vi "Backward Bracket Search.VI"(0 "string input with brackets":string) -> (1 "string start":string, 2 "string rest":string)   [LabVIEW 2010, in "NI_Gmath.lvlib"]
uses:
  NI_Gmath.lvlib
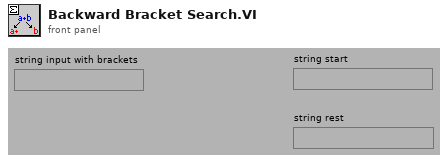
[diagram p1: front panel]
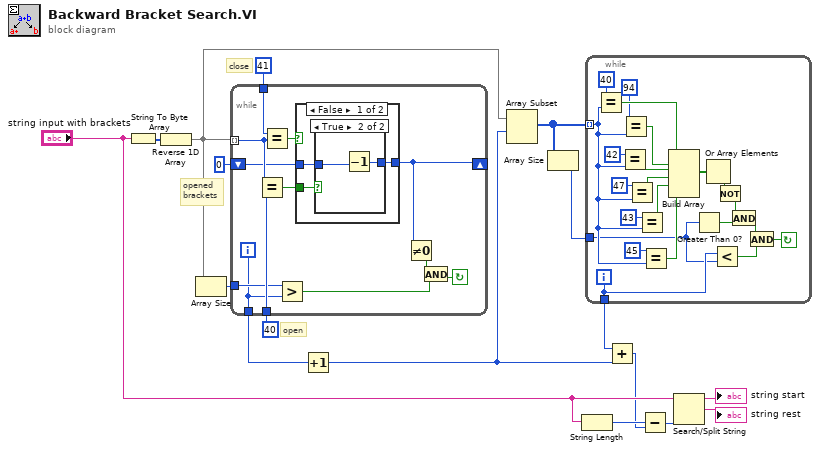
[diagram p0: block diagram]
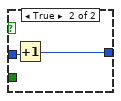
[diagram p3: hidden frame]
diagram:
  # "open"
  # "close"
  # "opened\nbrackets"
  n1 = String To Byte Array(string="string input with brackets") -> (unsigned byte array=w14:u8[])
  n2 = Reverse 1D Array(array=w14) -> (reversed array=w4:u8[])
  n3 = Array Size(array=w4) -> (size(s)=w13:i32)
  n4 = while {
    tunnel: [w18] -> w12
    tunnel: w13 -> [w23]
    tunnel: 40 -> [w27]
    tunnel: 41 -> [w29]
    tunnel: w4 -> [w26] mode=indexing
    shift-left: 0 -> [w20]
    shift-right: [w24] -> _
    i -> [w18]
    stop <- w21 continue-if-true
    n5 = Equal?(x=w26, y=w27) -> (x = y?=w25:bool)
    n6 = Equal?(x=w29, y=w26) -> (x = y?=w28:bool)
    n7 = Greater?(x=w23, y=w18) -> (0:w19:bool)
    n8 = case shown="False" w28 {
      tunnel: w20 -> [w31 w37]
      tunnel: [w30 w36] -> w24
      tunnel: w25 -> [w32 _]
      frame False {
        n9 = case shown="True" w32 {
          tunnel: w31 -> [w33 w35]
          tunnel: [w33 w34] -> w30
          frame False {
          }
          frame True {
            n10 = Decrement(x=w35) -> (x-1=w34:i32)
          }
        }
      }
      frame True {
        n11 = Increment(x=w37) -> (x+1=w36:i32)
      }
    }
    n12 = Not Equal To 0?(x=w24) -> (x != 0?=w22:bool)
    n13 = And(x=w22, y=w19) -> (x .and. y?=w21:bool)
  }
  n14 = Increment(x=w12) -> (x+1=w10:i32)
  n15 = Array Subset(array=w4, index=w10) -> (w1:u8[])  [unwired: 1 in]
  n16 = Array Size(array=w1) -> (size(s)=w2:i32)
  n17 = String Length(string="string input with brackets") -> (length=w8:i32)
  n18 = while {
    tunnel: w2 -> [w42]
    tunnel: [w45] -> w11
    tunnel: w1 -> [w59] mode=indexing
    i -> [w45]
    stop <- w39 continue-if-true
    n19 = Equal?(x=40, y=w59) -> (x = y?=w48:bool)
    n20 = Equal?(x=42, y=w59) -> (x = y?=w50:bool)
    n21 = Equal?(x=94, y=w59) -> (x = y?=w49:bool)
    n22 = Equal?(x=47, y=w59) -> (x = y?=w51:bool)
    n23 = Equal?(x=43, y=w59) -> (x = y?=w52:bool)
    n24 = Equal?(x=45, y=w59) -> (x = y?=w53:bool)
    n25 = Build Array(w48, w49, w50, w51, w52, w53) -> (w47:bool[])
    n26 = Greater Than 0?(x=w42) -> (x > 0?=w44:bool)
    n27 = Or Array Elements(Boolean array=w47) -> (logical OR=w46:bool)
    n28 = Less?(x=w45, y=w42) -> (x < y?=w41:bool)
    n29 = Not(x=w46) -> (.not. x?=w43:bool)
    n30 = And(x=w43, y=w44) -> (x .and. y?=w40:bool)
    n31 = And(x=w40, y=w41) -> (x .and. y?=w39:bool)
  }
  n32 = Add(x=w11, y=w10) -> (x+y=w7:i32)
  n33 = Subtract(x=w8, y=w7) -> (x-y=w6:i32)
  n34 = Search/Split String(string="string input with brackets", offset (0)=w6) -> (substring before match=→"string start":string, match + rest of string=→"string rest":string)  [unwired: 1 in, 1 out]
